vi "UDPReadTest.vi"() -> ()   [LabVIEW 2023]
panel:
  in  "stop":bool
  out "Pipeline Status":string
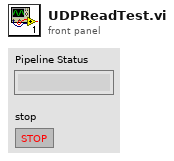
[diagram p1: front panel]
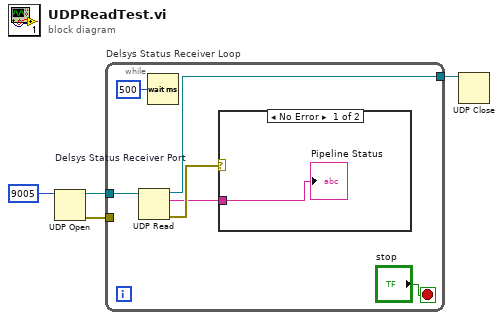
[diagram p0: block diagram]
diagram:
  n1 = UDP Open "Delsys Status Receiver Port"(11:9005) -> (port=w3:refnum<k16>, 0:w1:errorcluster)  [unwired: 4 in, 1 out]
  n2 = while "Delsys Status Receiver Loop" {
    tunnel: [w10] -> w4
    tunnel: w3 -> [w9]
    tunnel: w1 -> [_]
    stop <- "stop" stop-if-true
    n3 = UDP Read(connection ID=w9) -> (data out=w5:string, error out=w7:errorcluster, 3:w10:refnum<k16>)  [unwired: 3 in, 2 out]
    n4 = Wait (ms)(milliseconds to wait=500) -> ()  [unwired: 1 out]
    n5 = case shown="No Error" w7 {
      tunnel: w5 -> [w11 _]
      frame No Error {
        "Pipeline Status" <- w11
      }
      frame Error {
      }
    }
  }
  n6 = UDP Close(connection ID=w4) -> ()  [unwired: 1 in, 2 out]
